vi "refs_write_status_3.vi"(2 "error in":errorcluster, 3 "Value":string) -> (4 "error out":errorcluster)   [LabVIEW 2013]
uses:
  refs_var.vi
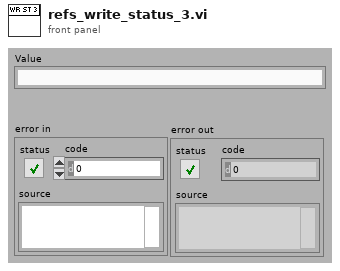
[diagram p1: front panel]
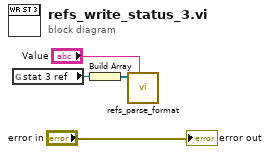
[diagram p0: block diagram]
diagram:
  n1 = global read "refs_var.vi" "stat 3 ref"() -> (w3:refnum<vi>)
  n2 = Build Array(w3) -> (w2:refnum<vi>[])
  n3 = call "refs_parse_format.vi"("string in"="Value", "str ind refs"=w2) -> ()  [unwired: 9 in, 1 out]
  "error out" <- "error in"
